vi "探头窗口-32-4列-服务器版.vi"() -> ()   [LabVIEW 2013]
panel:
  in  "外部停止命令？":bool=TRUE
  out "引用-探头属性[]":refnum<vi>
  out "引用-监测模式？":refnum<vi>
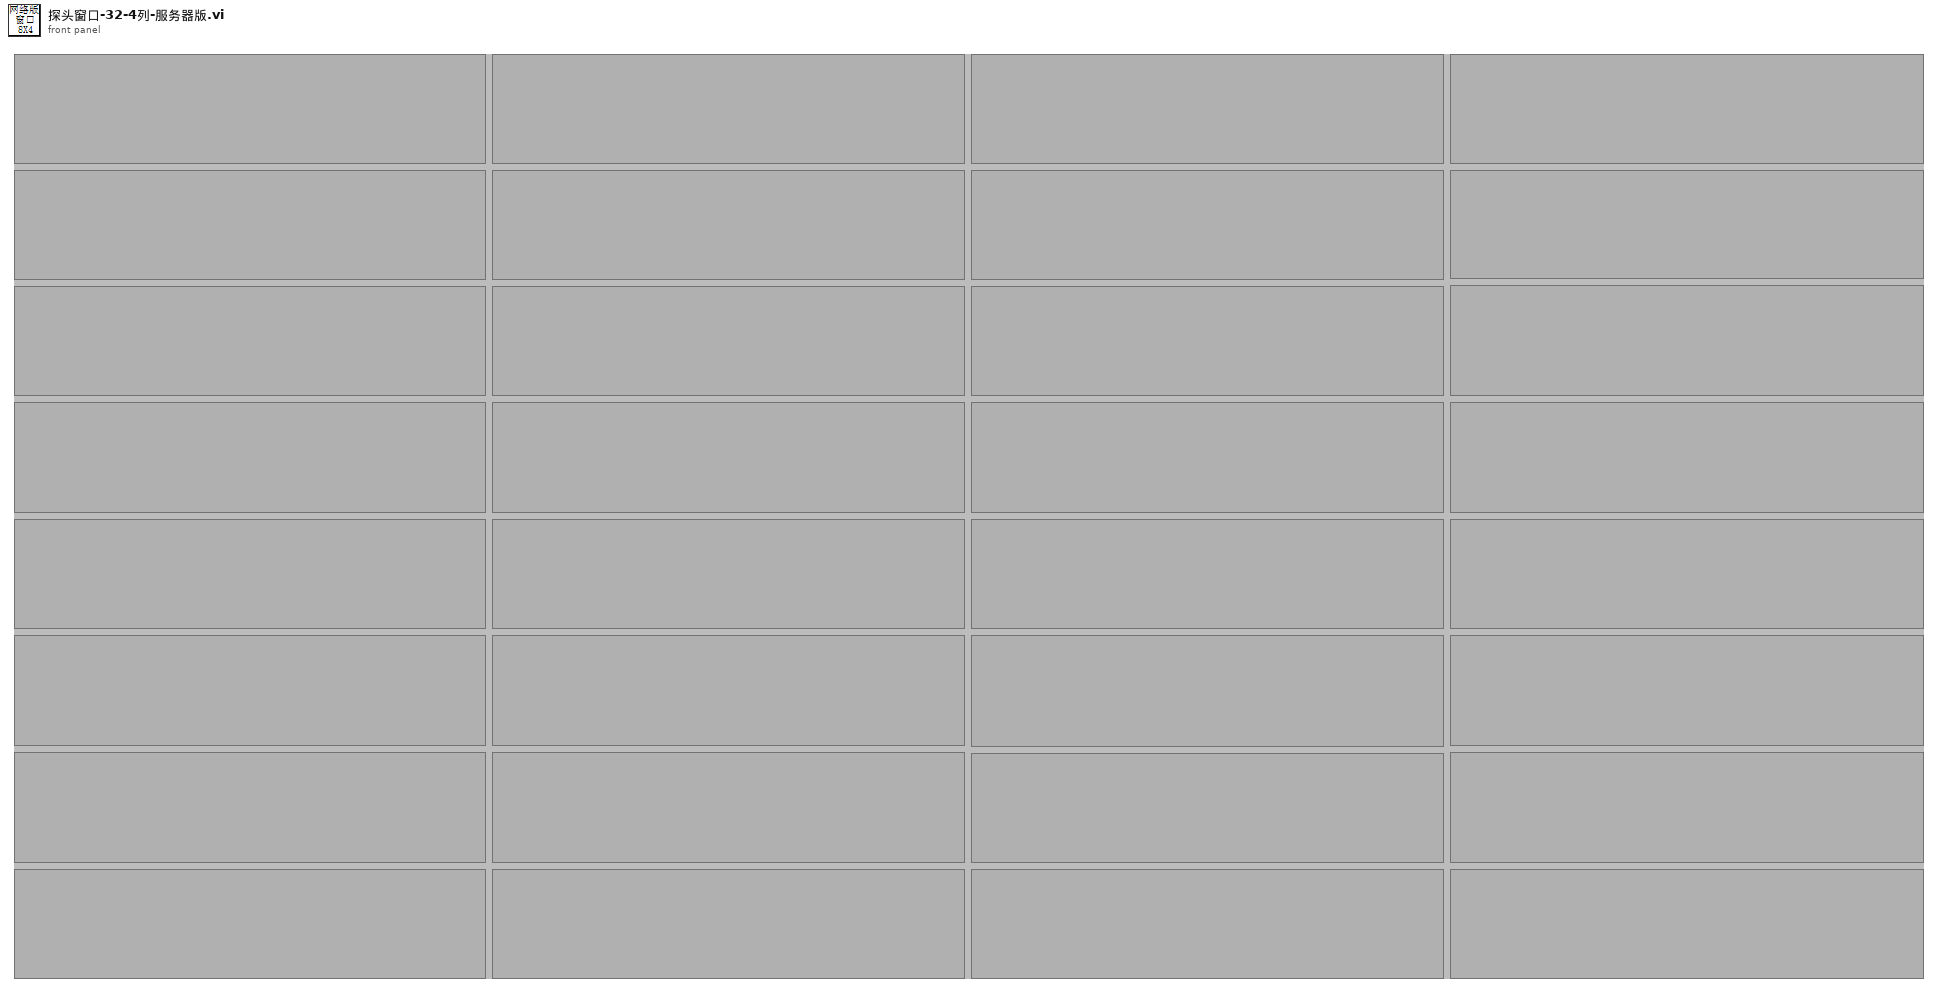
[diagram p1: front panel]
types:
  T1 = typedef "eventvkey.ctl" = enum16{"ASCII", "Enter", "Return", "Shift", "Ctrl", "Alt", "Cmd", "Opt", "Caps", "NumLock", "Clear", "Break", "Up", "Down", "Left", "Right", "Insert", "Delete", "Home", "End", "PageUp", "PageDown", "Escape", "Help", "Pause", "ScrollLock", "F1", "F2", "F3", "F4", "F5", "F6", "F7", "F8", "F9", "F10", "F11", "F12", "F13", "F14", "F15", "F16", "F17", "F18", "F19", "F20", "F21", "F22", "F23", "F24", "Play", "VolumeUp", "VolumeDown", "Mute", "Two Byte Char"}
  T2 = cluster{"探头地址与信息":cluster{"网络地址":cluster{"IP":string, "port":u16}, "探头信息":string}, "测量值":cluster{"时间":timestamp, "数值":dbl}, "限值":cluster{"限值1":dbl, "限值2":dbl}, "探头状态":enum16{"正常", "离线", "禁用", "一级报警", "二级报警"}}[]
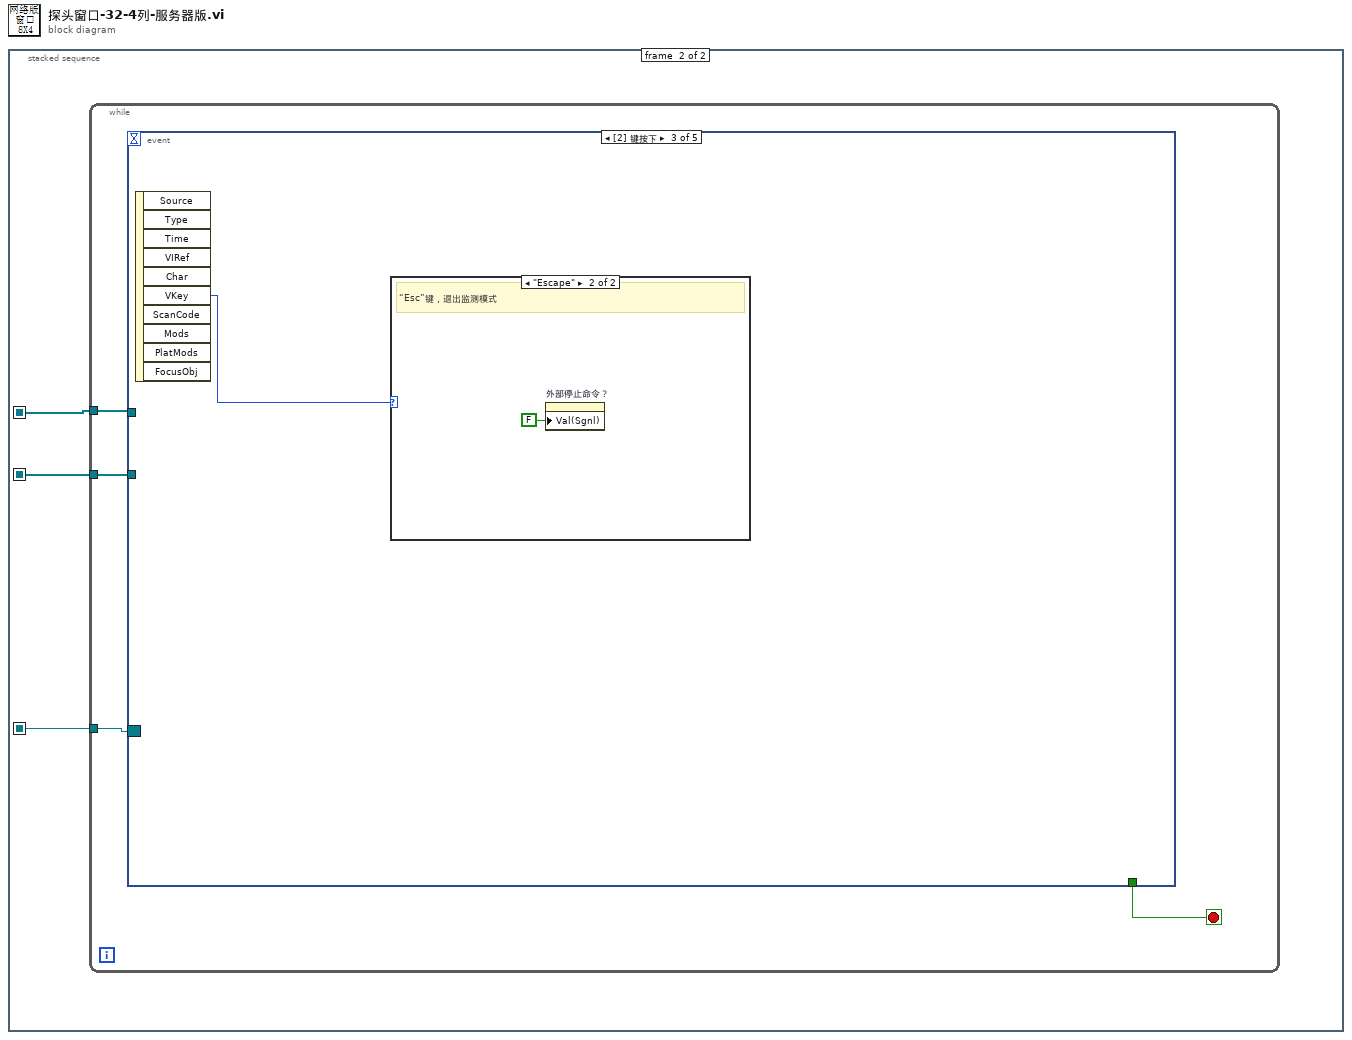
[diagram p0: block diagram]
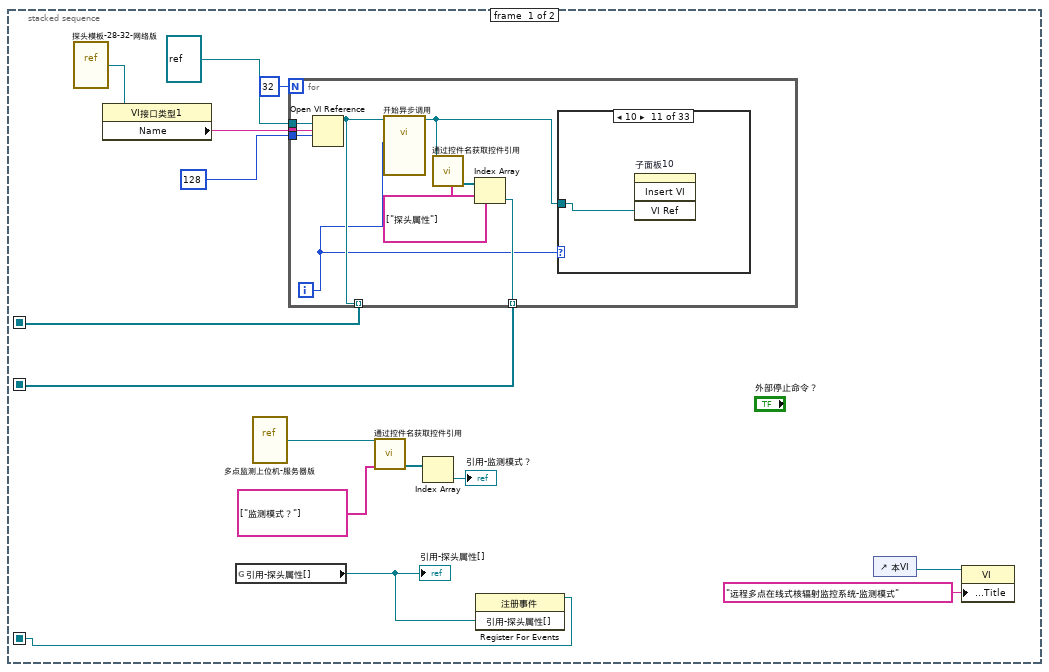
[diagram p2: hidden frame]
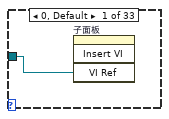
[diagram p3: hidden frame]
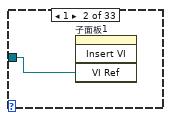
[diagram p4: hidden frame]
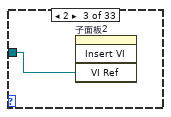
[diagram p5: hidden frame]
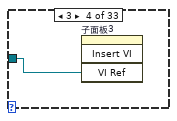
[diagram p6: hidden frame]
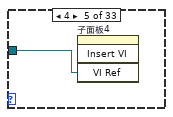
[diagram p7: hidden frame]
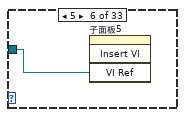
[diagram p8: hidden frame]
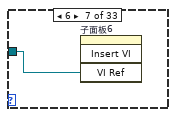
[diagram p9: hidden frame]
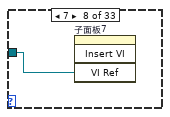
[diagram p10: hidden frame]
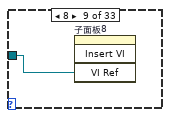
[diagram p11: hidden frame]
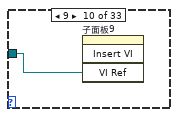
[diagram p12: hidden frame]
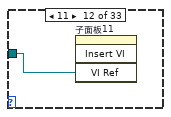
[diagram p13: hidden frame]
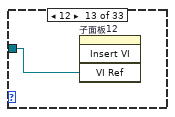
[diagram p14: hidden frame]
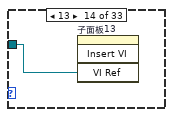
[diagram p15: hidden frame]
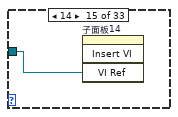
[diagram p16: hidden frame]
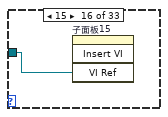
[diagram p17: hidden frame]
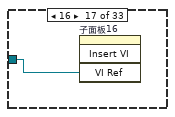
[diagram p18: hidden frame]
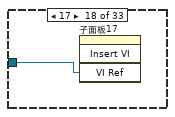
[diagram p19: hidden frame]
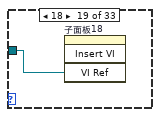
[diagram p20: hidden frame]
diagram:
  n1 = stacked-sequence {
    seq-local: [w10 _] -> [_ w59]
    seq-local: [w9 _] -> [_ w58]
    seq-local: [w3 _] -> [_ w57]
    frame #0 {
      n2 = vi-ref "探头模板-28-32-网络版.vi"() -> (w15:refnum<vi>)
      n3 = property class="VI接口类型1"(reference=w15) -> ("Name"=w14:string)  [unwired: 1 in, 2 out]
      n4 = global read "全局变量-35点监测.vi" "引用-探头属性[]"() -> (w4:refnum<vi>)
      "引用-探头属性[]" <- w4
      n5 = vi-ref "多点监测上位机-服务器版.vi"() -> (w8:refnum<vi>)
      n6 = for {
        N: 32 -> [_]
        tunnel: w14 -> [w24]
        tunnel: 128 ("选项") -> [w23]
        tunnel: refnum<vi> refnum ("类型说明符VI引用句柄（仅用于类型）") -> [w22]
        tunnel: [w18] -> w10 mode=indexing
        tunnel: [w19] -> w9 mode=indexing
        i -> [w16]
        n7 = Open VI Reference(type specifier VI Refnum (for type only)=w22, vi path=w24, options=w23) -> (vi reference=w18:refnum<vi>)  [unwired: 3 in, 1 out]
        n8 = call-by-ref "开始异步调用"(reference=w18, "探头序号"=w16) -> (reference out=w17:refnum<vi>)  [unwired: 12 in, 1 out]
        n9 = call "通过控件名获取控件引用.vi"("控件名数组"=string[] ["探头属性"], "VI引用"=w17) -> ("控件引用输出"=w20:refnum<vi>[])  [unwired: 7 in, 2 out]
        n10 = Index Array(array=w20) -> (element=w19:refnum<vi>)  [unwired: 1 in]
        n11 = case shown="10" w16 {
          tunnel: w17 -> [w25 w26 w27 w28 w29 w30 w31 w32 w33 w34 w35 w36 w37 w38 w39 w40 w41 w42 w43 w44 w45 w46 w47 w48 w49 w50 w51 w52 w53 w54 w55 w56 _]
          frame 0, Default {
            n12 = invoke on="子面板" class="子面板" method="Insert VI"("VI Ref"=w25) -> ()  [unwired: 3 in, 4 out]
          }
          frame 1 {
            n13 = invoke on="子面板1" class="SubPnl" method="Insert VI"("VI Ref"=w26) -> ()  [unwired: 3 in, 4 out]
          }
          frame 2 {
            n14 = invoke on="子面板2" class="SubPnl" method="Insert VI"("VI Ref"=w27) -> ()  [unwired: 3 in, 4 out]
          }
          frame 3 {
            n15 = invoke on="子面板3" class="SubPnl" method="Insert VI"("VI Ref"=w28) -> ()  [unwired: 3 in, 4 out]
          }
          frame 4 {
            n16 = invoke on="子面板4" class="SubPnl" method="Insert VI"("VI Ref"=w29) -> ()  [unwired: 3 in, 4 out]
          }
          frame 5 {
            n17 = invoke on="子面板5" class="SubPnl" method="Insert VI"("VI Ref"=w30) -> ()  [unwired: 3 in, 4 out]
          }
          frame 6 {
            n18 = invoke on="子面板6" class="SubPnl" method="Insert VI"("VI Ref"=w31) -> ()  [unwired: 3 in, 4 out]
          }
          frame 7 {
            n19 = invoke on="子面板7" class="SubPnl" method="Insert VI"("VI Ref"=w32) -> ()  [unwired: 3 in, 4 out]
          }
          frame 8 {
            n20 = invoke on="子面板8" class="SubPnl" method="Insert VI"("VI Ref"=w33) -> ()  [unwired: 3 in, 4 out]
          }
          frame 9 {
            n21 = invoke on="子面板9" class="SubPnl" method="Insert VI"("VI Ref"=w34) -> ()  [unwired: 3 in, 4 out]
          }
          frame 10 {
            n22 = invoke on="子面板10" class="SubPnl" method="Insert VI"("VI Ref"=w35) -> ()  [unwired: 3 in, 4 out]
          }
          frame 11 {
            n23 = invoke on="子面板11" class="SubPnl" method="Insert VI"("VI Ref"=w36) -> ()  [unwired: 3 in, 4 out]
          }
          frame 12 {
            n24 = invoke on="子面板12" class="SubPnl" method="Insert VI"("VI Ref"=w37) -> ()  [unwired: 3 in, 4 out]
          }
          frame 13 {
            n25 = invoke on="子面板13" class="SubPnl" method="Insert VI"("VI Ref"=w38) -> ()  [unwired: 3 in, 4 out]
          }
          frame 14 {
            n26 = invoke on="子面板14" class="SubPnl" method="Insert VI"("VI Ref"=w39) -> ()  [unwired: 3 in, 4 out]
          }
          frame 15 {
            n27 = invoke on="子面板15" class="SubPnl" method="Insert VI"("VI Ref"=w40) -> ()  [unwired: 3 in, 4 out]
          }
          frame 16 {
            n28 = invoke on="子面板16" class="SubPnl" method="Insert VI"("VI Ref"=w41) -> ()  [unwired: 3 in, 4 out]
          }
          frame 17 {
            n29 = invoke on="子面板17" class="SubPnl" method="Insert VI"("VI Ref"=w42) -> ()  [unwired: 3 in, 4 out]
          }
          frame 18 {
            n30 = invoke on="子面板18" class="SubPnl" method="Insert VI"("VI Ref"=w43) -> ()  [unwired: 3 in, 4 out]
          }
          frame 19 {
            n31 = invoke on="子面板19" class="SubPnl" method="Insert VI"("VI Ref"=w44) -> ()  [unwired: 3 in, 4 out]
          }
          frame 20 {
            n32 = invoke on="子面板20" class="SubPnl" method="Insert VI"("VI Ref"=w45) -> ()  [unwired: 3 in, 4 out]
          }
          frame 21 {
            n33 = invoke on="子面板21" class="SubPnl" method="Insert VI"("VI Ref"=w46) -> ()  [unwired: 3 in, 4 out]
          }
          frame 22 {
            n34 = invoke on="子面板22" class="SubPnl" method="Insert VI"("VI Ref"=w47) -> ()  [unwired: 3 in, 4 out]
          }
          frame 23 {
            n35 = invoke on="子面板23" class="SubPnl" method="Insert VI"("VI Ref"=w48) -> ()  [unwired: 3 in, 4 out]
          }
          frame 24 {
            n36 = invoke on="子面板24" class="SubPnl" method="Insert VI"("VI Ref"=w49) -> ()  [unwired: 3 in, 4 out]
          }
          frame 25 {
            n37 = invoke on="子面板25" class="SubPnl" method="Insert VI"("VI Ref"=w50) -> ()  [unwired: 3 in, 4 out]
          }
          frame 26 {
            n38 = invoke on="子面板26" class="SubPnl" method="Insert VI"("VI Ref"=w51) -> ()  [unwired: 3 in, 4 out]
          }
          frame 27 {
            n39 = invoke on="子面板27" class="SubPnl" method="Insert VI"("VI Ref"=w52) -> ()  [unwired: 3 in, 4 out]
          }
          frame 28 {
            n40 = invoke on="子面板28" class="SubPnl" method="Insert VI"("VI Ref"=w53) -> ()  [unwired: 3 in, 4 out]
          }
          frame 29 {
            n41 = invoke on="子面板29" class="SubPnl" method="Insert VI"("VI Ref"=w54) -> ()  [unwired: 3 in, 4 out]
          }
          frame 30 {
            n42 = invoke on="子面板30" class="SubPnl" method="Insert VI"("VI Ref"=w55) -> ()  [unwired: 3 in, 4 out]
          }
          frame 31 {
            n43 = invoke on="子面板31" class="SubPnl" method="Insert VI"("VI Ref"=w56) -> ()  [unwired: 3 in, 4 out]
          }
          frame 32 {
          }
        }
      }
      n44 = call "通过控件名获取控件引用.vi"("控件名数组"=string[] ["监测模式？"], "VI引用"=w8) -> ("控件引用输出"=w6:refnum<vi>[])  [unwired: 7 in, 2 out]
      n45 = Index Array(array=w6) -> (element=→"引用-监测模式？":refnum<vi>)  [unwired: 1 in]
      n46 = register-events(w4) -> (reference out=w3:refnum<event-registration>)  [unwired: 2 in, 1 out]
      n47 = control-ref of="本VI"() -> (w2:refnum<vi>)
      n48 = property class="VI"(reference=w2, "Front Panel.Title"="远程多点在线式核辐射监控系统-监测模式" ("前面板窗口:标题")) -> ()  [unwired: 1 in, 2 out]
    }
    frame #1 {
      n49 = while {
        tunnel: w59 -> [w62]
        tunnel: w58 -> [w61]
        tunnel: w57 -> [w60]
        stop <- w63 stop-if-true
        n50 = event shown="[2] 键按下" {
          selector: w60 -> [_ _ _ w68 _]
          dyn-events: _ -> [_ _ _ _ _]
          timeout: _ -> [_ _ _ _ _]
          tunnel: [_ _ _ TRUE ("放弃？") _] -> w63
          tunnel: w62 -> [_ _ _ w70 _]
          tunnel: w61 -> [_ _ _ _ w86]
          event Timeout {
            n51 = event-data() -> ()  [unwired: 1 in, 3 out]
          }
          event Panel Close? {
            n52 = event-data() -> ()  [unwired: 1 in, 4 out]
            n53 = property on="外部停止命令？" class="Bool (严格)"("Val(Sgnl)"=FALSE ("值(信号)")) -> ()  [unwired: 2 in, 2 out]
            n54 = event-data("Discard?"=TRUE ("放弃？")) -> ()  [unwired: 1 in, 1 out]
          }
          event Key Down {
            n55 = event-data() -> ("VKey"=w66:T1)  [unwired: 1 in, 9 out]
            n56 = case shown="\"Escape\"" w66 {
              frame "ASCII", Default {
              }
              frame "Escape" {
                # "“Esc”键，退出监测模式"
                n57 = property on="外部停止命令？" class="Bool (严格)"("Val(Sgnl)"=FALSE ("值(信号)")) -> ()  [unwired: 2 in, 2 out]
              }
            }
          }
          event "外部停止命令？": Value Change {
            # "注销事件，防止“探头属性值改变”事件自动触发 ，导致前面板锁定"
            n58 = event-data() -> ()  [unwired: 1 in, 6 out]
            n59 = flat-sequence {
              tunnel: w70 -> [w73]
              tunnel: [w73] -> w69
              tunnel: w68 -> [w72]
              tunnel: w69 -> [w80]
              frame #0 {
                n60 = Unregister For Events(event registration refnum=w72) -> ()  [unwired: 1 in, 1 out]
              }
              frame #1 {
                w79 = FALSE  # F
                n61 = for {
                  tunnel: w80 -> [w85] mode=indexing
                  tunnel: [w81] -> w76
                  n62 = invoke class="VI (严格)" method="Abort VI"(reference=w85) -> (reference out=w83:refnum<vi>, error out=w84:errorcluster)  [unwired: 2 in, 1 out]
                  n63 = Close Reference(reference=w83, error in (no error)=w84) -> (error out=w82:errorcluster)
                  n64 = call <vilib>:"Clear Errors.vi"("error in (no error)"=w82) -> ("error out"=w81:errorcluster)  [unwired: 6 in]
                }
                n65 = local read "引用-监测模式？"() -> (w78:refnum<vi>)
                n66 = control-ref of="本VI"() -> (w77:refnum<vi>)
                n67 = property class="Ctl"(reference=w78, error in=w76, "Val(Sgnl)"=w79) -> (error out=w75:errorcluster)  [unwired: 1 out]
                n68 = invoke class="VI" method="FP.Close"(reference=w77, error in=w75) -> (error out=w74:errorcluster)  [unwired: 1 in, 2 out]
                n69 = call <vilib>:"Clear Errors.vi"("error in (no error)"=w74) -> ()  [unwired: 6 in, 1 out]
              }
            }
          }
          event Value Change {
            n70 = event-data() -> ("NewVal"=w87:T2)  [unwired: 1 in, 5 out]
            n71 = for {
              workers-P: _ -> [_]
              tunnel: w86 -> [w89] mode=indexing
              tunnel: w87 -> [w88] mode=indexing
              # "各个“探头属性”赋值（信号）"
              n72 = property class="Ctl"(reference=w89, "Val(Sgnl)"=w88) -> ()  [unwired: 1 in, 2 out]
            }
          }
        }
      }
    }
  }
